vi "Write ConnectConfig.vi"(8 "error in (no error)":errorcluster, 10 "ConnectConfig":T1={"IP Address"="", "Port"=102, "Timeout"=5000}, 11 "PLC_Module in":refnum<class "PLC_Module.lvclass">) -> (0 "error out":errorcluster, 3 "PLC_Module out":refnum<class "PLC_Module.lvclass">)   [LabVIEW 2025, in "PLC_Module.lvlib" / "PLC_Module.lvclass"]
uses:
  PLC_Module.lvclass
  PLC_Module.lvclass/PLC_Module.ctl
  PLC_Connect_Config.ctl
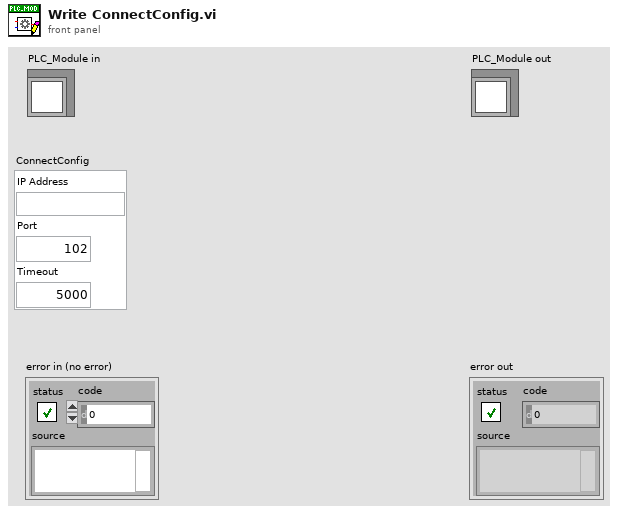
[diagram p1: front panel]
types:
  T1 = typedef "PLC_Module.lvlib/PLC_Module.lvclass/PLC_Connect_Config.ctl" = cluster{"IP Address":string, "Port":u16, "Timeout":i32}
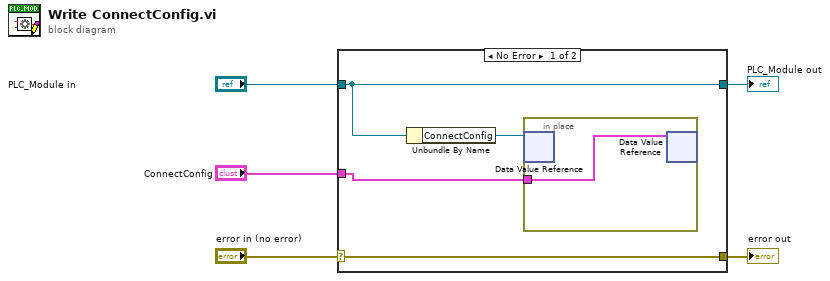
[diagram p0: block diagram]
diagram:
  n1 = case shown="No Error" "error in (no error)" {
    selector: "error in (no error)" -> [w9 w11]
    tunnel: [w9 w11] -> w4
    tunnel: [w8 w12] -> w2
    tunnel: "PLC_Module in" -> [w8 w12]
    tunnel: "ConnectConfig" -> [w6 _]
    frame No Error {
      n2 = Unbundle By Name(w8) -> ("ConnectConfig"=w7:refnum<data-value>)
      n3 = in-place {
        in-place-border: w6 -> [w10]
        n4 = in-place-dvr #1(w7) -> ()  [unwired: 2 out]
        n5 = in-place-dvr #1(w10) -> ()  [unwired: 2 out]
      }
    }
    frame Error {
    }
  }
  "error out" <- w4
  "PLC_Module out" <- w2
